vi "prime and composite,and evenand odd.vi"() -> ()   [LabVIEW 2018]
panel:
  out "odd":i32[](array[numeric])
  out "even":i32[](array[numeric])
  out "composite number":i32[](array[numeric])
  out "prime number":i32[](array[numeric])
  in  "Numeric":dbl
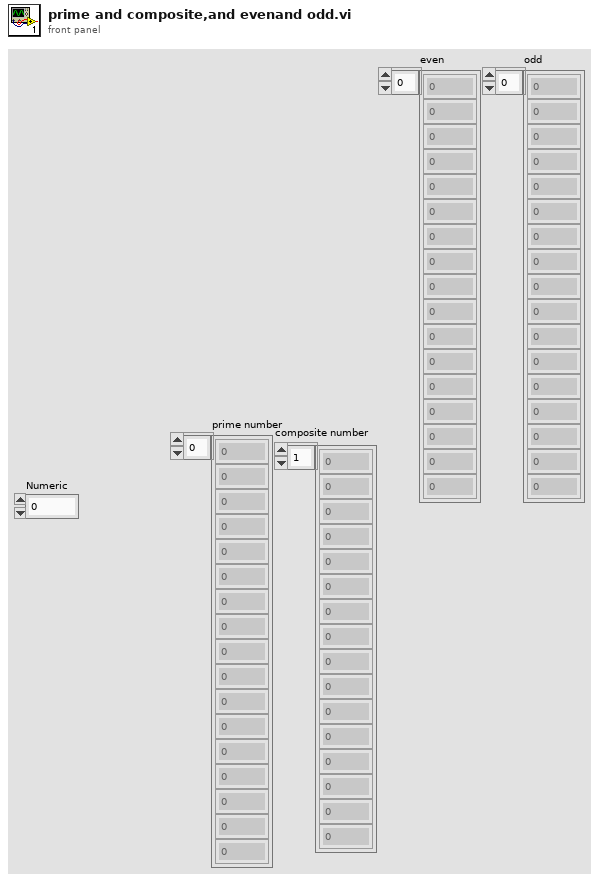
[diagram p1: front panel]
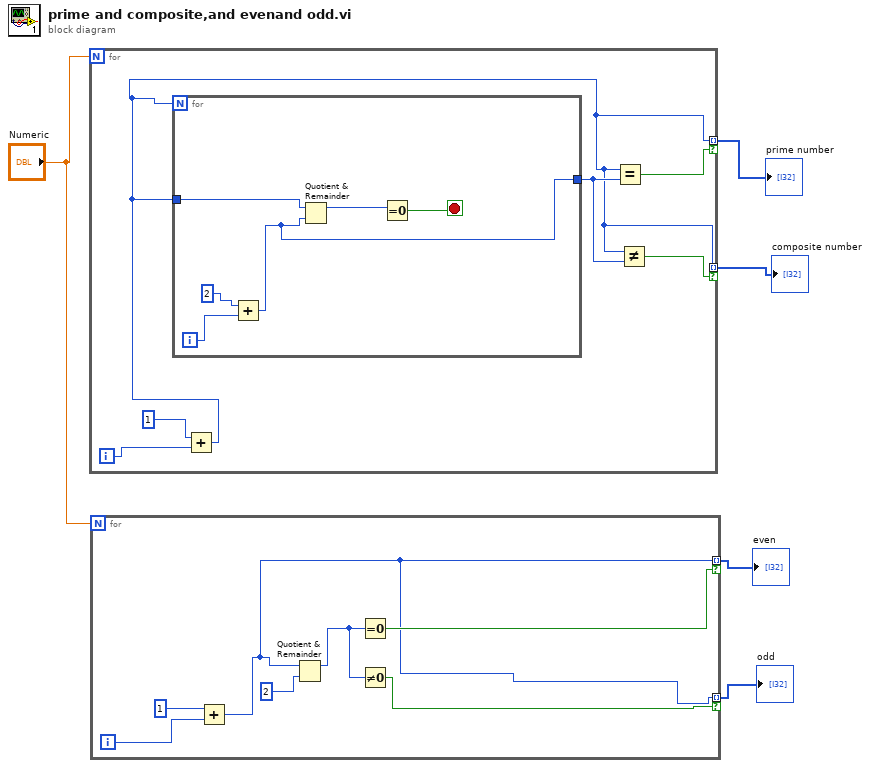
[diagram p0: block diagram]
diagram:
  n1 = for {
    N: "Numeric" -> [_]
    tunnel: [w7] -> w5 mode=indexing if=w8
    tunnel: [w7] -> w4 mode=indexing if=w6
    i -> [w11]
    n2 = Add(x=1, y=w11) -> (x+y=w7:i32)
    n3 = for {
      N: w7 -> [_]
      tunnel: w7 -> [w15]
      tunnel: [w14] -> w9
      i -> [w17]
      stop <- w12 stop-if-true
      n4 = Add(x=2, y=w17) -> (x+y=w14:i32)
      n5 = Quotient & Remainder(x=w15, y=w14) -> (x-y*floor(x/y)=w13:i32)  [unwired: 1 out]
      n6 = Equal To 0?(x=w13) -> (x = 0?=w12:bool)
    }
    n7 = Equal?(x=w7, y=w9) -> (x = y?=w8:bool)
    n8 = Not Equal?(x=w7, y=w9) -> (x != y?=w6:bool)
  }
  "prime number" <- w5
  "composite number" <- w4
  n9 = for {
    N: "Numeric" -> [_]
    tunnel: [w20] -> w2 mode=indexing if=w21
    tunnel: [w20] -> w1 mode=indexing if=w19
    i -> [w24]
    n10 = Add(x=1, y=w24) -> (x+y=w20:i32)
    n11 = Quotient & Remainder(x=w20, y=2) -> (x-y*floor(x/y)=w18:i32)  [unwired: 1 out]
    n12 = Equal To 0?(x=w18) -> (x = 0?=w21:bool)
    n13 = Not Equal To 0?(x=w18) -> (x != 0?=w19:bool)
  }
  "even" <- w2
  "odd" <- w1
